vi "find control ref.vi"(8 "error in":errorcluster, 10 "Control Name":string, 11 "Controls[]":refnum<vi>[](array[refnum])) -> (0 "error out":errorcluster, 2 "Control Found":bool, 3 "Control refout":refnum<vi>)   [LabVIEW 2016, in "sub-VIs.lvlib"]
uses:
  sub-VIs.lvlib
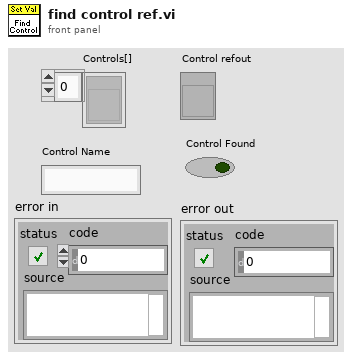
[diagram p1: front panel]
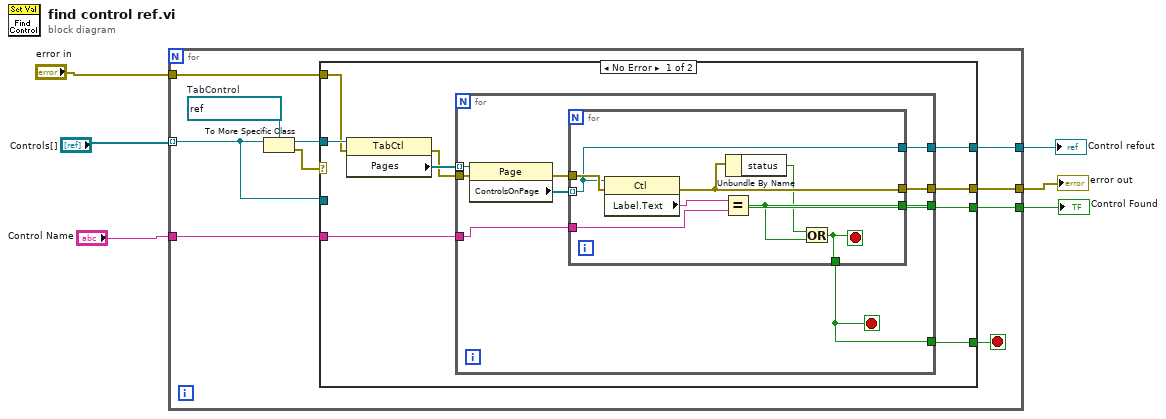
[diagram p0: block diagram]
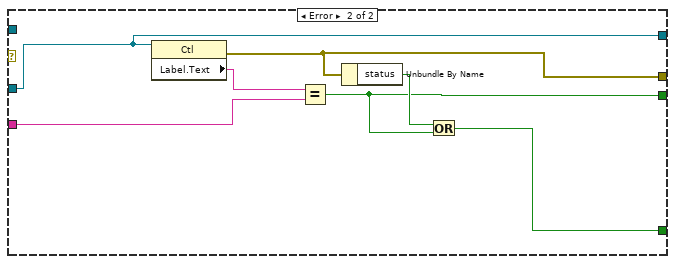
[diagram p2: hidden frame]
diagram:
  n1 = for {
    tunnel: "Controls[]" -> [w12] mode=indexing
    tunnel: [w14] -> w4
    tunnel: "Control Name" -> [w11]
    tunnel: [w10] -> w5
    tunnel: [w8] -> w6
    tunnel: "error in" -> [w7]
    stop <- w9 stop-if-true
    w16 = refnum<vi> refnum  # TabControl
    n2 = To More Specific Class(target class=w16, reference=w12) -> (specific class reference=w15:refnum<vi>, error out=w13:errorcluster)  [unwired: 1 in]
    n3 = case shown="No Error" w13 {
      tunnel: w15 -> [w25 _]
      tunnel: [w23 w45] -> w14
      tunnel: w12 -> [_ w43]
      tunnel: w11 -> [w22 w48]
      tunnel: [w20 w47] -> w10
      tunnel: [w19 w44] -> w9
      tunnel: [w18 w43] -> w8
      tunnel: w7 -> [w17 _]
      frame No Error {
        n4 = property class="TabCtl"(reference=w25, error in=w17) -> (error out=w21:errorcluster, "Pages"=w24:refnum<vi>[])  [unwired: 1 out]
        n5 = for {
          tunnel: w24 -> [w34] mode=indexing
          tunnel: [w33] -> w23
          tunnel: w22 -> [w31]
          tunnel: w21 -> [w30]
          tunnel: [w28] -> w20
          tunnel: [w27] -> w19
          tunnel: [w26] -> w18
          stop <- w27 stop-if-true
          n6 = property class="Page"(reference=w34, error in=w30) -> (error out=w29:errorcluster, "ControlsOnPage"=w32:refnum<vi>[])  [unwired: 1 out]
          n7 = for {
            tunnel: w32 -> [w35] mode=indexing
            tunnel: [w38] -> w33
            tunnel: w31 -> [w41]
            tunnel: w29 -> [w40]
            tunnel: [w39] -> w28
            tunnel: [w36] -> w27
            tunnel: [w35] -> w26
            stop <- w36 stop-if-true
            n8 = property class="Ctl"(reference=w35, error in=w40) -> (error out=w39:errorcluster, "Label.Text"=w42:string)  [unwired: 1 out]
            n9 = Equal?(x=w42, y=w41) -> (x = y?=w38:bool)
            n10 = Unbundle By Name(w39) -> ("status"=w37:bool)
            n11 = Or(x=w37, y=w38) -> (x .or. y?=w36:bool)
          }
        }
      }
      frame Error {
        n12 = property class="Ctl"(reference=w43) -> (error out=w47:errorcluster, "Label.Text"=w49:string)  [unwired: 1 in, 1 out]
        n13 = Equal?(x=w49, y=w48) -> (x = y?=w45:bool)
        n14 = Unbundle By Name(w47) -> ("status"=w46:bool)
        n15 = Or(x=w46, y=w45) -> (x .or. y?=w44:bool)
      }
    }
  }
  "Control refout" <- w6
  "error out" <- w5
  "Control Found" <- w4
